vi "Demo_Grab.vi"() -> ()   [LabVIEW 2024]
doc: "Grab any video source supported by QuickTime (internal, USB, FW, etc).\nThe output image can be compressed with any QT supported format (See image->compressed_data).\nSet Dialogs to 1 in Frame grabber settings to use the standard QT dialog.\n\nChris Salzmann © 1994-2003"
uses:
  <userlib>/ImageProcessing/QTLIB_2595_LV86/QT_Private.ctl
  <userlib>/ImageProcessing/QTLIB_2595_LV86/QT_Video.ctl
  <userlib>/ImageProcessing/QTLIB_2595_LV86/QT_Compression.ctl
  <userlib>/ImageProcessing/QTLIB_2595_LV86/QT_FrameGrabber.ctl
panel:
  in  "Case Constant\n(See Context Help)":bool=TRUE
  in  "Compression":i32(slide)=745 scale=0.0..1024.0 scale format="%x"
  in  "Codec (raw )":T1(ring)=enum."jpeg"
  out "error out":errorcluster
  in  "White l.":dbl(slide)=80.61224489795919 scale=0.0..100.0
  in  "Black l.":dbl(slide)=14.285714285714286 scale=0.0..100.0
  in  "Sharp":dbl(slide)=1.7857142857142858 scale=0.0..100.0
  in  "Contr":dbl(slide)=53.57142857142858 scale=0.0..100.0
  in  "Bright":dbl(slide)=53.06122448979592 scale=0.0..100.0
  in  "Sat":dbl(slide)=51.02040816326531 scale=0.0..100.0
  in  "Hue":dbl(slide)=50.0 scale=0.0..100.0
  out "CIN info":string="© Chris 94-2002, QT Fat-CIN, rev: 2528, FATQTCin.c, May 29 2002, 21:48:22"
  out "QT Version":string="QuickTime v. 502 "
  out "Picture":picture
  in  "stop":bool
  in  "Frame Grabber Settings":T2={"Name"="", "Digitizer"=2, "Input"=1, "Width"=160, "Height"=120, "Input format"=enum."NTSC", "Frame rate"=0.0, "Reserved"=0, "Dialogs"=0} {"Frame rate" format="%#1_6g"; "Dialogs" format="%.0b"}
  # "Grab any video source supported by QuickTime (internal, USB, FW, etc).\nThe output image can be compressed with any QT supported format (See image->compressed_data).\nSet Dialogs to 1 in Frame grabber settings to use the standard QT dialog.\n\nChris Salzmann © 1994-2008"
  # "No compression\n-> raw"
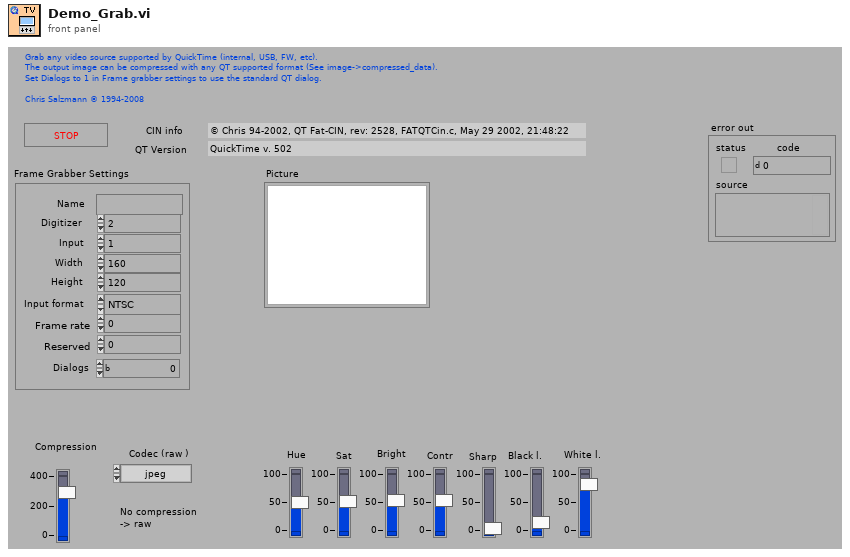
[diagram p1: front panel]
types:
  T1 = enum16{"rle ", "WRLE", "cvid", "yuv2", "dvcp", "dvc ", "dvpp", "smc ", "h261", "h263", "mjp2", "mjpa", "mjpb", "mp4v", "raw ", "VP31", "jpeg", "8BPS", "png ", "SVQ1", "SVQ3", "tga ", "tiff", "rpza", "ZyGo"}
  T2 = typedef "QT_FrameGrabber.ctl" = cluster{"Name":string, "Digitizer":i32, "Input":i32, "Width":i32, "Height":i32, "Input format":enum32{"NTSC", "PAL", "Secam"}, "Frame rate":dbl, "Reserved":i32, "Dialogs":u32}
  T3 = typedef "QT_Compression.ctl" = cluster{"Compression":i32, "Format":i32, "Codec":i32, "Comp. Quality":i32, "Key Frame":i32, "Dialogs":u32}
  T4 = typedef "QT_Video.ctl" = cluster{"Color format":u32, "Hue":dbl, "Saturation":dbl, "Brightness":dbl, "Contrast":dbl, "Sharpness":dbl, "Black Level":dbl, "White Level":dbl, "Options":i32, "Dialogs":u32}
  T5 = typedef "QT_Private.ctl" = cluster{"reserved 1":i32, "reserved 2":i32, "reserved 3":i32, "reserved 4":i32}
  T6 = typedef "QT_Ref.ctl" = refnum<k1>
  T7 = typedef "QT_Image.ctl" = cluster{"Width":i32, "Height":i32, "Depth":i32, "data":u8[], "Compressed data":u8[], "Color table":u32[], "Duration":i32, "Options":i32, "Timestamp":i32, "ID":i32, "Reserved":i32, "Dialogs":u32}
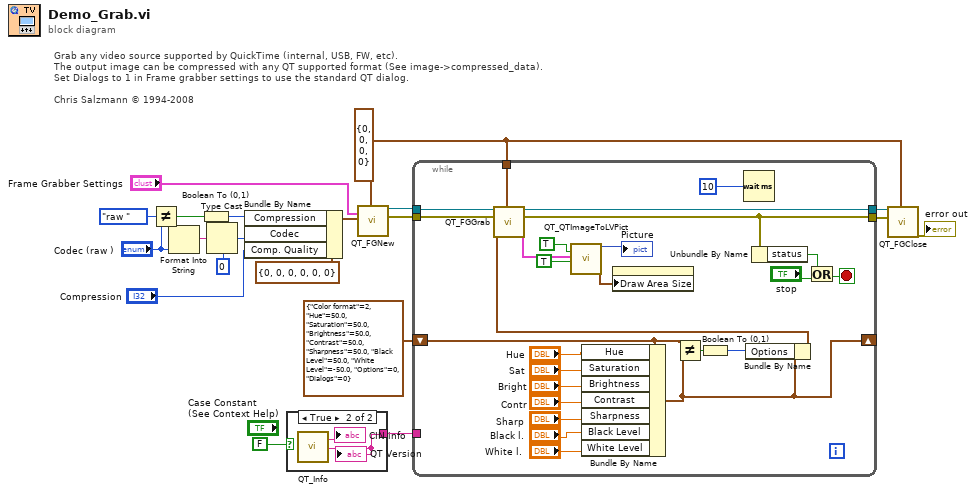
[diagram p0: block diagram]
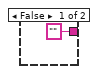
[diagram p2: hidden frame]
diagram:
  w7 = T5 {"reserved 1"=0, "reserved 2"=0, "reserved 3"=0, "reserved 4"=0} ("Private")
  # "Grab any video source supported by QuickTime (internal, USB, FW, etc).\nThe output image can be compressed with any QT supported format (See image->compressed_data).\nSet Dialogs to 1 in Frame grabber settings to use the standard QT dialog.\n\nChris Salzmann © 1994-2008"
  n1 = Not Equal?(x=T1."raw " ("codec (raw )"), y="Codec (raw )") -> (x != y?=w3:bool)
  n2 = Format Into String("Codec (raw )") -> (resulting string=w12:string)  [unwired: 3 in, 1 out]
  n3 = Boolean To (0,1)(Boolean=w3) -> (0, 1=w2:i16)
  n4 = Type Cast(type=0 ("Codec"), x=w12) -> (*(type *) &x=w11:i32)
  n5 = Bundle By Name(cluster=T3 {"Compression"=0, "Format"=0, "Codec"=0, "Comp. Quality"=0, "Key Frame"=0, "Dialogs"=0} ("Compression Settings"), "Compression"=w2, "Codec"=w11, "Comp. Quality"="Compression") -> (w13:T3)
  n6 = case shown="True" FALSE {
    tunnel: ["" ("QT Version") w23] -> w6
    frame False {
    }
    frame True {
      n7 = call <userlib>:"QT_Info.vi"() -> ("CIN info"=→"CIN info":string, "QT Version"=w23:string)  [unwired: 3 in, 15 out]
      "QT Version" <- w23
    }
  }
  n8 = call <userlib>:"QT_FGNew.vi"("Frame Grabber Settings"="Frame Grabber Settings", "Compression Settings"=w13, "Private"=w7) -> ("QT Ref Out"=w19:T6, "error out"=w15:errorcluster)  [unwired: 2 in, 13 out]
  n9 = while {
    shift-left: T4 {"Color format"=2, "Hue"=50.0, "Saturation"=50.0, "Brightness"=50.0, "Contrast"=50.0, "Sharpness"=50.0, "Black Level"=50.0, "White Level"=-50.0, "Options"=0, "Dialogs"=0} ("Video Settings") -> [w33]
    shift-right: [w31] -> _
    tunnel: [w44] -> w17
    tunnel: w15 -> [w45]
    tunnel: w7 -> [w46]
    tunnel: [w48] -> w20
    tunnel: w19 -> [w49]
    tunnel: w6 -> [_]
    stop <- w43 stop-if-true
    n10 = Bundle By Name(cluster=w33, "Hue"="Hue", "Saturation"="Sat", "Brightness"="Bright", "Contrast"="Contr", "Sharpness"="Sharp", "Black Level"="Black l.", "White Level"="White l.") -> (w31:T4)
    n11 = Not Equal?(x=w33, y=w31) -> (x != y?=w32:bool)
    n12 = Boolean To (0,1)(Boolean=w32) -> (0, 1=w25:i16)
    n13 = Wait (ms)(milliseconds to wait=u32 10) -> ()  [unwired: 1 out]
    n14 = Bundle By Name(cluster=w31, "Options"=w25) -> (w30:T4)
    n15 = call <userlib>:"QT_FGGrab.vi"("QT Ref In"=w49, "Video Settings in"=w30, "error in (no error)"=w45, "Private"=w46) -> ("QT Ref Out"=w48:T6, "Image/Movie Out"=w29:T7, "error out"=w44:errorcluster)  [unwired: 2 in, 11 out]
    n16 = call <userlib>:"QT_QTImageToLVPict.vi"("Draw info"=TRUE, "Image/Movie Out"=w29, "BW image"=TRUE) -> ("Picture color"=→"Picture":picture, "Pict Draw Area Size"=w26:cluster{"Width":i16, "Height":i16})  [unwired: 15 out]
    n17 = property on="Picture" class="Pict"("Draw Area Size"=w26) -> ()  [unwired: 2 in, 2 out]
    n18 = Unbundle By Name(w44) -> ("status"=w41:bool)
    n19 = Or(x=w41, y="stop") -> (x .or. y?=w43:bool)
  }
  n20 = call <userlib>:"QT_FGClose.vi"("QT Ref In"=w20, "error in (no error)"=w17, "Private"=w7) -> ("error out"=→"error out":errorcluster)  [unwired: 1 in, 15 out]
